vi "Ref AVI Video Initialise.vi"(8 "error in (no error)":errorcluster, 9 "Channel":T1=enum."Green Channel", 11 "Timelapse folder path":path) -> (0 "error out":errorcluster)   [LabVIEW 2020]
uses:
  Typedefs/Channel Selector.ctl
  Typedefs/AVI Refs cluster.ctl
  <vilib>/vision/Avi.llb/IMAQ AVI2 Refnum.ctl
  <vilib>/vision/Image Controls.llb/IMAQ Image.ctl
  <vilib>/vision/Avi1.llb/AviRefnum.ctl
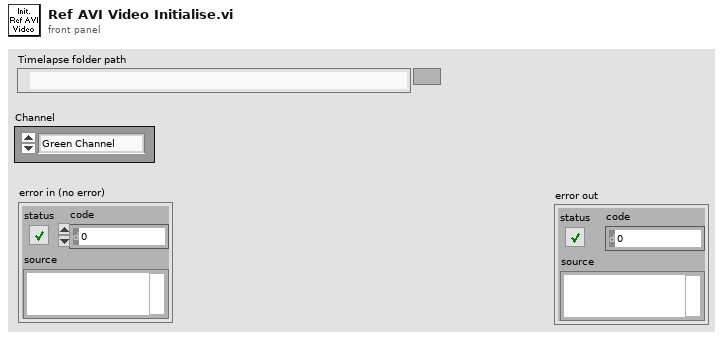
[diagram p1: front panel]
types:
  T1 = typedef "Channel Selector.ctl" = enum16{"Red Channel", "Green Channel", "Blended"}
  T2 = typedef "AVI Refs cluster.ctl" = cluster{"AVI2 path":path, "AVI 2 Refnum":T3, "New Image":T4, "error out":errorcluster, "Avi 1 Refnum":T5}
  T3 = typedef "IMAQ AVI2 Refnum.ctl" = refnum<k20>
  T4 = typedef "IMAQ Image.ctl" = refnum<image>
  T5 = typedef "AviRefnum.ctl" = refnum<k1>
  T6 = enum16{"Write Red AVI", "Write Green AVI", "Write AVI mode"}
  T7 = typedef "Image Type" = u32
  T8 = typedef "AVI implementation enum.ctl" = enum16{"AVI1", "AVI2"}
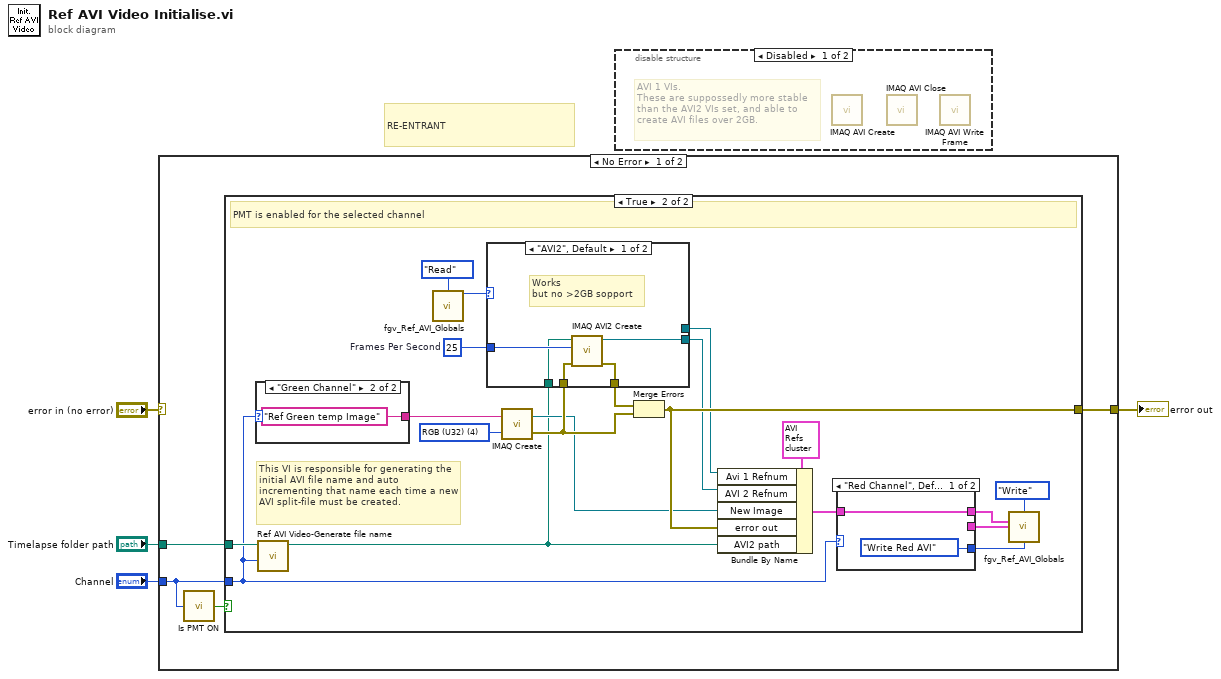
[diagram p0: block diagram]
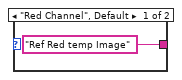
[diagram p4: hidden frame]
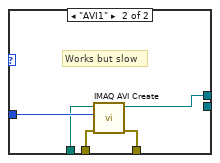
[diagram p5: hidden frame]
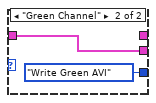
[diagram p6: hidden frame]
diagram:
  # "RE-ENTRANT"
  n1 = case shown="No Error" "error in (no error)" {
    selector: "error in (no error)" -> [_ w45]
    tunnel: "Timelapse folder path" -> [w8 _]
    tunnel: "Channel" -> [w6 _]
    tunnel: [w7 w45] -> w2
    frame No Error {
      n2 = call "Is PMT ON.vi"("Channel"=w6) -> ("PMT is ON"=w5:bool)
      n3 = case shown="True" w5 {
        tunnel: w8 -> [_ w28]
        tunnel: w6 -> [_ w9]
        tunnel: [_ w22] -> w7
        frame False {
          # "Channel not used / PMT control = 0"
        }
        frame True {
          w26 = u32 25  # Frames Per Second
          w27 = T7 4 items=["Grayscale (U8)", "Grayscale (I16)", "Grayscale (SGL)", "Complex (CSG)", "RGB (U32)", "HSL (U32)", "RGB (U64)", "Grayscale (U16)"] ("Image Type")
          # "This VI is responsible for generating the initial AVI file name and auto incrementing that name each time a new AVI split-file must be created."
          # "PMT is enabled for the selected channel"
          n4 = case shown="\"Green Channel\"" w9 {
            tunnel: ["Ref Red temp Image" ("Image Name") "Ref Green temp Image" ("Image Name")] -> w10
            frame "Red Channel", Default {
            }
            frame "Green Channel" {
            }
          }
          n5 = call "Ref AVI Video-Generate file name.vi"("Channel"=w9, "Videos folder path"=w28) -> ("AVI file path & name"=w11:path)  [unwired: 8 in, 1 out]
          n6 = call "fgv_Ref_AVI_Globals.vi"("Function"=enum16{"Intialize", "Write", "Read", "Clear"}."Read") -> ("AVI mode"=w16:T8)  [unwired: 11 in, 3 out]
          n7 = call "IMAQ Create"("Image Name"=w10, "Image Type"=w27) -> ("New Image"=w21:T4, "error out"=w25:errorcluster)  [unwired: 2 in, 1 out]
          n8 = case shown="\"AVI2\", Default" w16 {
            tunnel: w26 -> [w35 w40]
            tunnel: w11 -> [w34 w39]
            tunnel: w25 -> [w33 w38]
            tunnel: [w32 w37] -> w24
            tunnel: [w31 _] -> w20
            tunnel: [_ w36] -> w18
            frame "AVI2", Default {
              # "Works\nbut no >2GB sopport"
              n9 = call "IMAQ AVI2 Create"("error in (no error)"=w33, "Frames Per Second"=w35, "AVI Path"=w34) -> ("error out"=w32:errorcluster, "AVI Refnum"=w31:T3)  [unwired: 7 in]
            }
            frame "AVI1" {
              # "Works but slow"
              n10 = call "IMAQ AVI Create"("error in (no error)"=w38, "Frames Per Second"=w40, "AVI Path"=w39) -> ("error out"=w37:errorcluster, "Avi Refnum"=w36:T5)  [unwired: 7 in]
            }
          }
          n11 = Merge Errors(w24, w25) -> (w22:errorcluster)
          n12 = Bundle By Name(cluster=T2 {"AVI2 path"=path "", "AVI 2 Refnum"=refnum, "New Image"=refnum, "error out"={"status"=FALSE, "code"=0, "source"=""}, "Avi 1 Refnum"=refnum} ("Green AVI"), "Avi 1 Refnum"=w18, "AVI 2 Refnum"=w20, "New Image"=w21, "error out"=w22, "AVI2 path"=w11) -> (w19:T2)
          n13 = case shown="\"Red Channel\", Default" w9 {
            tunnel: w19 -> [w41 w44]
            tunnel: [_ w44] -> w14
            tunnel: [T6."Write Red AVI" ("\"Write\" sub function") T6."Write Green AVI" ("\"Write\" sub function")] -> w13
            tunnel: [w41 _] -> w12
            frame "Red Channel", Default {
            }
            frame "Green Channel" {
            }
          }
          n14 = call "fgv_Ref_AVI_Globals.vi"("Function"=enum16{"Intialize", "Write", "Read", "Clear"}."Write", "Red Ref AVI"=w12, "Green Ref AVI"=w14, "\"Write\" sub function"=w13) -> ()  [unwired: 8 in, 4 out]
        }
      }
    }
    frame Error {
    }
  }
  "error out" <- w2
  n15 = disable-structure shown="Disabled" {
    frame Disabled {
      # "AVI 1 VIs.\nThese are suppossedly more stable\nthan the AVI2 VIs set, and able to\ncreate AVI files over 2GB."
      n16 = call "IMAQ AVI Create"() -> ()  [unwired: 10 in, 2 out]
      n17 = call "IMAQ AVI Close"() -> ()  [unwired: 11 in, 1 out]
      n18 = call "IMAQ AVI Write Frame"() -> ()  [unwired: 10 in, 2 out]
    }
    frame Enabled {
    }
  }
